vi "Set Server Stop UE.vi"(10 "Server Stop UE":refnum<user-event>, 11 "OOP Server in":refnum<class "HVC.lvclass">) -> (3 "OOP Server out":refnum<class "HVC.lvclass">)   [LabVIEW 2019, in "HVC.lvlib" / "HVC.lvclass"]
uses:
  HVC.lvclass
  HVC.lvclass/HVC.ctl
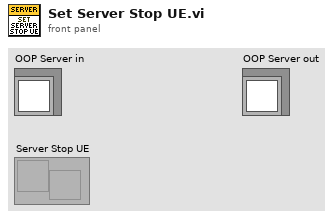
[diagram p1: front panel]
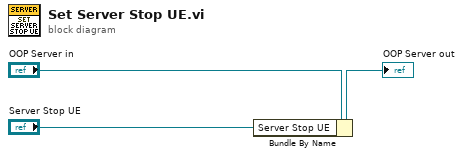
[diagram p0: block diagram]
diagram:
  n1 = Bundle By Name(cluster="OOP Server in", "Server Stop UE"="Server Stop UE") -> (→"OOP Server out":refnum<class "HVC.lvclass">)
